vi "ecg_ncs_v8_67.vi"() -> ()   [LabVIEW 2016]
uses:
  <instrlib>/niUSRP/niUSRP Timestamp.ctl
  C:/Program Files/National Instruments/LabVIEW 2016/examples/Instrument IO/Serial/support/Serial - Settings.ctl
  State.ctl
  <vilib>/Instr/_visa.llb/VISA Configure Serial Port (Instr).vi
  <instrlib>/niUSRP/niUSRP Fetch Rx Data (2D CDB).vi
  <instrlib>/niUSRP/niUSRP Write Tx Data (2D CDB).vi
panel:
  out "size(s) 3":i32
  out "AmpNcsDSLast":dbl[](array[numeric])
  in  "Low-Pass Freq":dbl=200.0 format="%#_13g"
  in  "Wait  ECG":i32=1
  in  "max queue size":i32=-1
  in  "Wait NCS":i32=-1
  out "ECG time":u32
  out "NCS time":u32
  in  "File Name 3":string="Test2"
  out "size(s) 4":i32
  in  "maxWrite 2":i32=2000
  out "AmpNcs":dbl[](array[numeric])
  out "PhNcs":dbl[](array[numeric])
  in  "Sampling Rate":i32=500
  out "AmpNcsDS":dbl[](array[numeric])
  out "PhNcsDS":dbl[](array[numeric])
  in  "Tab Control 3":enum32{"ECG Sample", "ECG"}(tab)
  out "?":i32(graph)
  out "?":i16(graph)
  in  "maxWrite":i32=2000
  out "size(s) 2":i32
  out "sizeNcsDS":i32
  in  "File Name":string="freq2G_1"
  in  "Path":path=path "D:/Research/SummerFall17Spring18/CnC/NCS/EcgNcsCorrelation/CodeAndData/Data/Mar03"
  out "#Loop = #Packets Received":i32
  out "ECGsample":i16
  out "error IO 2":errorcluster={"status"=FALSE, "code"=-1074118647, "source"=""}
  in  "Serial Settings":T1={"baud rate"=57600, "data bits"=8, "parity"=enum."None", "stop bits"=10, "flow control"=0} {"flow control" items=["None"=0, "XON/XOFF"=1, "RTS/CTS"=2, "DTR/DSR"=4]; "stop bits" items=["1.0"=10, "1.5"=15, "2.0"=20]; "data bits" min=5 max=8 step=1; "baud rate" items=["75"=75, "110"=110, "134"=134, "150"=150, "300"=300, "600"=600, "1200"=1200, "1800"=1800, "2400"=2400, "4800"=4800, "7200"=7200, "9600"=9600, "14400"=14400, "19200"=19200, "28800"=28800, "38400"=38400, "56000"=56000, "57600"=57600, "115200"=115200, "128000"=128000, "230400"=230400]}
  in  "VISA resource name":refnum<visa-resource-name>="bmd101"
  in  "byte count":u32=1
  out "Coerced Rx IQ Rate":dbl
  out "Gain":dbl=-15.0
  out "Bandwidth":dbl=56000000.0
  out "Coerced Carrier Frequency":dbl=2000000000.0 format="%#.17g"
  out "Coerced Tx IQ rate":dbl=1000000.0
  out "error IO":errorcluster={"status"=FALSE, "code"=-1074118647, "source"=""}
  in  "Rx Number of Samples":i32=10000
  in  "Tab Control 2":enum32{"NI-294x/295x", "NI-2900/2901"}(tab)=enum."NI-2900/2901"
  in  "Rx carrier frequency [Hz]":dbl=2000000000.0 format="%#_6p"
  in  "Tx carrier frequency [Hz]":dbl=1000000000.0 format="%#_6p"
  in  "Start Trigger Time":T2={"whole seconds"=1, "fractional seconds"=0.0}
  in  "Tab Control":T3(tab)
  out "?":dbl[](graph)
  out "NCS Amp Chart":dbl[](graph)=[0.011967714738528729, 0.012021355192189592, 0.012015275039596582, 0.011969166030167903, 0.011958890166168242, 0.012007893820858737, 0.012022893722444085, 0.011978222225113794, 0.011969989939463181, 0.012003099640895068]
  out "NCS Phase Chart":dbl[](graph)=[0.011967714738528729, 0.012021355192189592, 0.012015275039596582, 0.011969166030167903, 0.011958890166168242, 0.012007893820858737, 0.012022893722444085, 0.011978222225113794, 0.011969989939463181, 0.012003099640895068]
  out "Tx Waveform Graph":waveform(dbl)[](graph)
  in  "Stop":bool
  in  "Tone Amplitude":dbl=0.707 step=0.05 format="%#.6g"
  in  "Tone  Frequency":dbl=5000.0 format="%#_6p"
  in  "Tx Waveform Size":dbl=2000.0
  in  "Device Name":refnum<k15>="MyB210"
  in  "Tx Gain":dbl=28.0 format="%#_6f"
  in  "Tx IQ Rate":dbl=1000000.0 format="%#_6p"
  in  "Rx Gain":dbl=32.0 format="%#_6f"
  in  "Rx IQ Rate":dbl=1000000.0 format="%#_6p"
  # "Rx Settings"
  # "Tx Settings"
  # "Note that on the NI-2900 and NI-2901, both Rx channels share an LO and both Tx channels share an LO. However, on the NI-294x/295x devices, Rx and Tx of channel 0 share an LO and Rx and Tx of channel 1 share an LO."
  # "Rx: Number of samples should be 1e6/512 in one loop."
  # "This Tx graph should always have end and start tied up since this is being sent in a loop continuously. Otherwise phase jumps will be noticed."
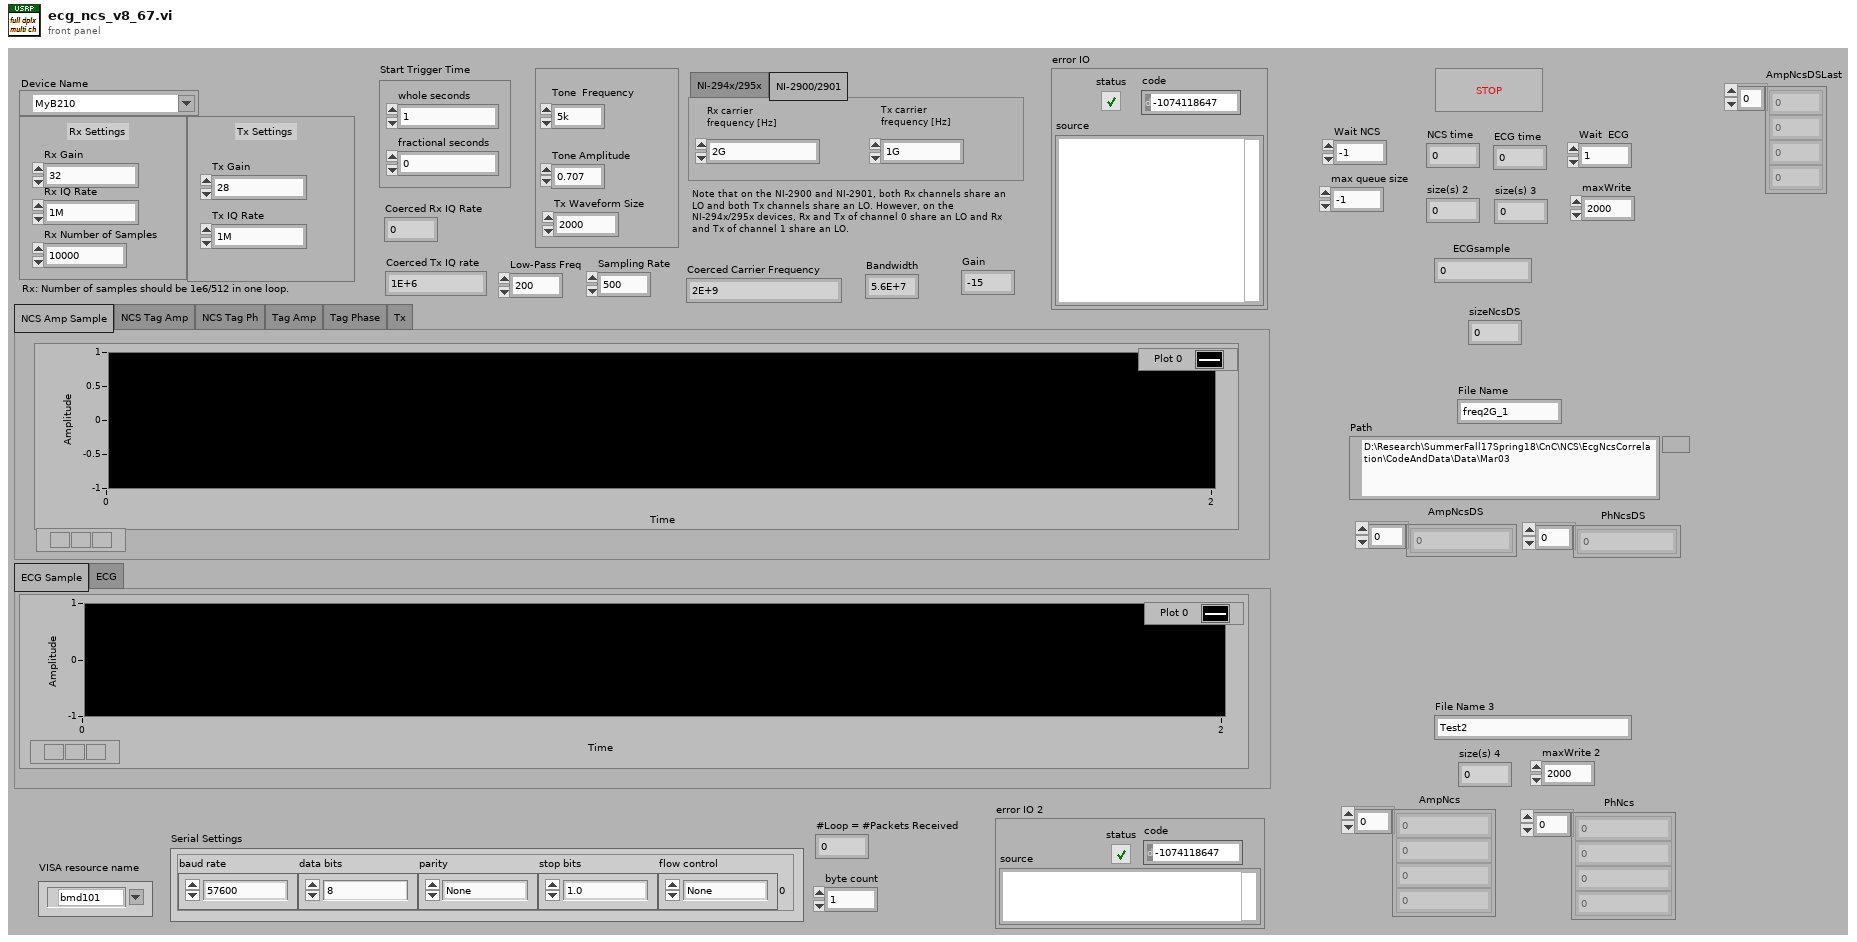
[diagram p1: front panel]
types:
  T1 = typedef "Serial - Settings.ctl" = cluster{"baud rate":u32, "data bits":u16, "parity":enum16{"None", "Odd", "Even", "Mark", "Space"}, "stop bits":u16, "flow control":u16}
  T2 = typedef "niUSRP Timestamp.ctl" = cluster{"whole seconds":u64, "fractional seconds":dbl}
  T3 = enum32{"NCS Amp Sample", "NCS Tag Amp", "NCS Tag Ph", "Tag Amp", "Tag Phase", "Tx"}
  T4 = typedef "State.ctl" = enum16{"Initialize", "get byte", "check", "packet received", "packet approved"}
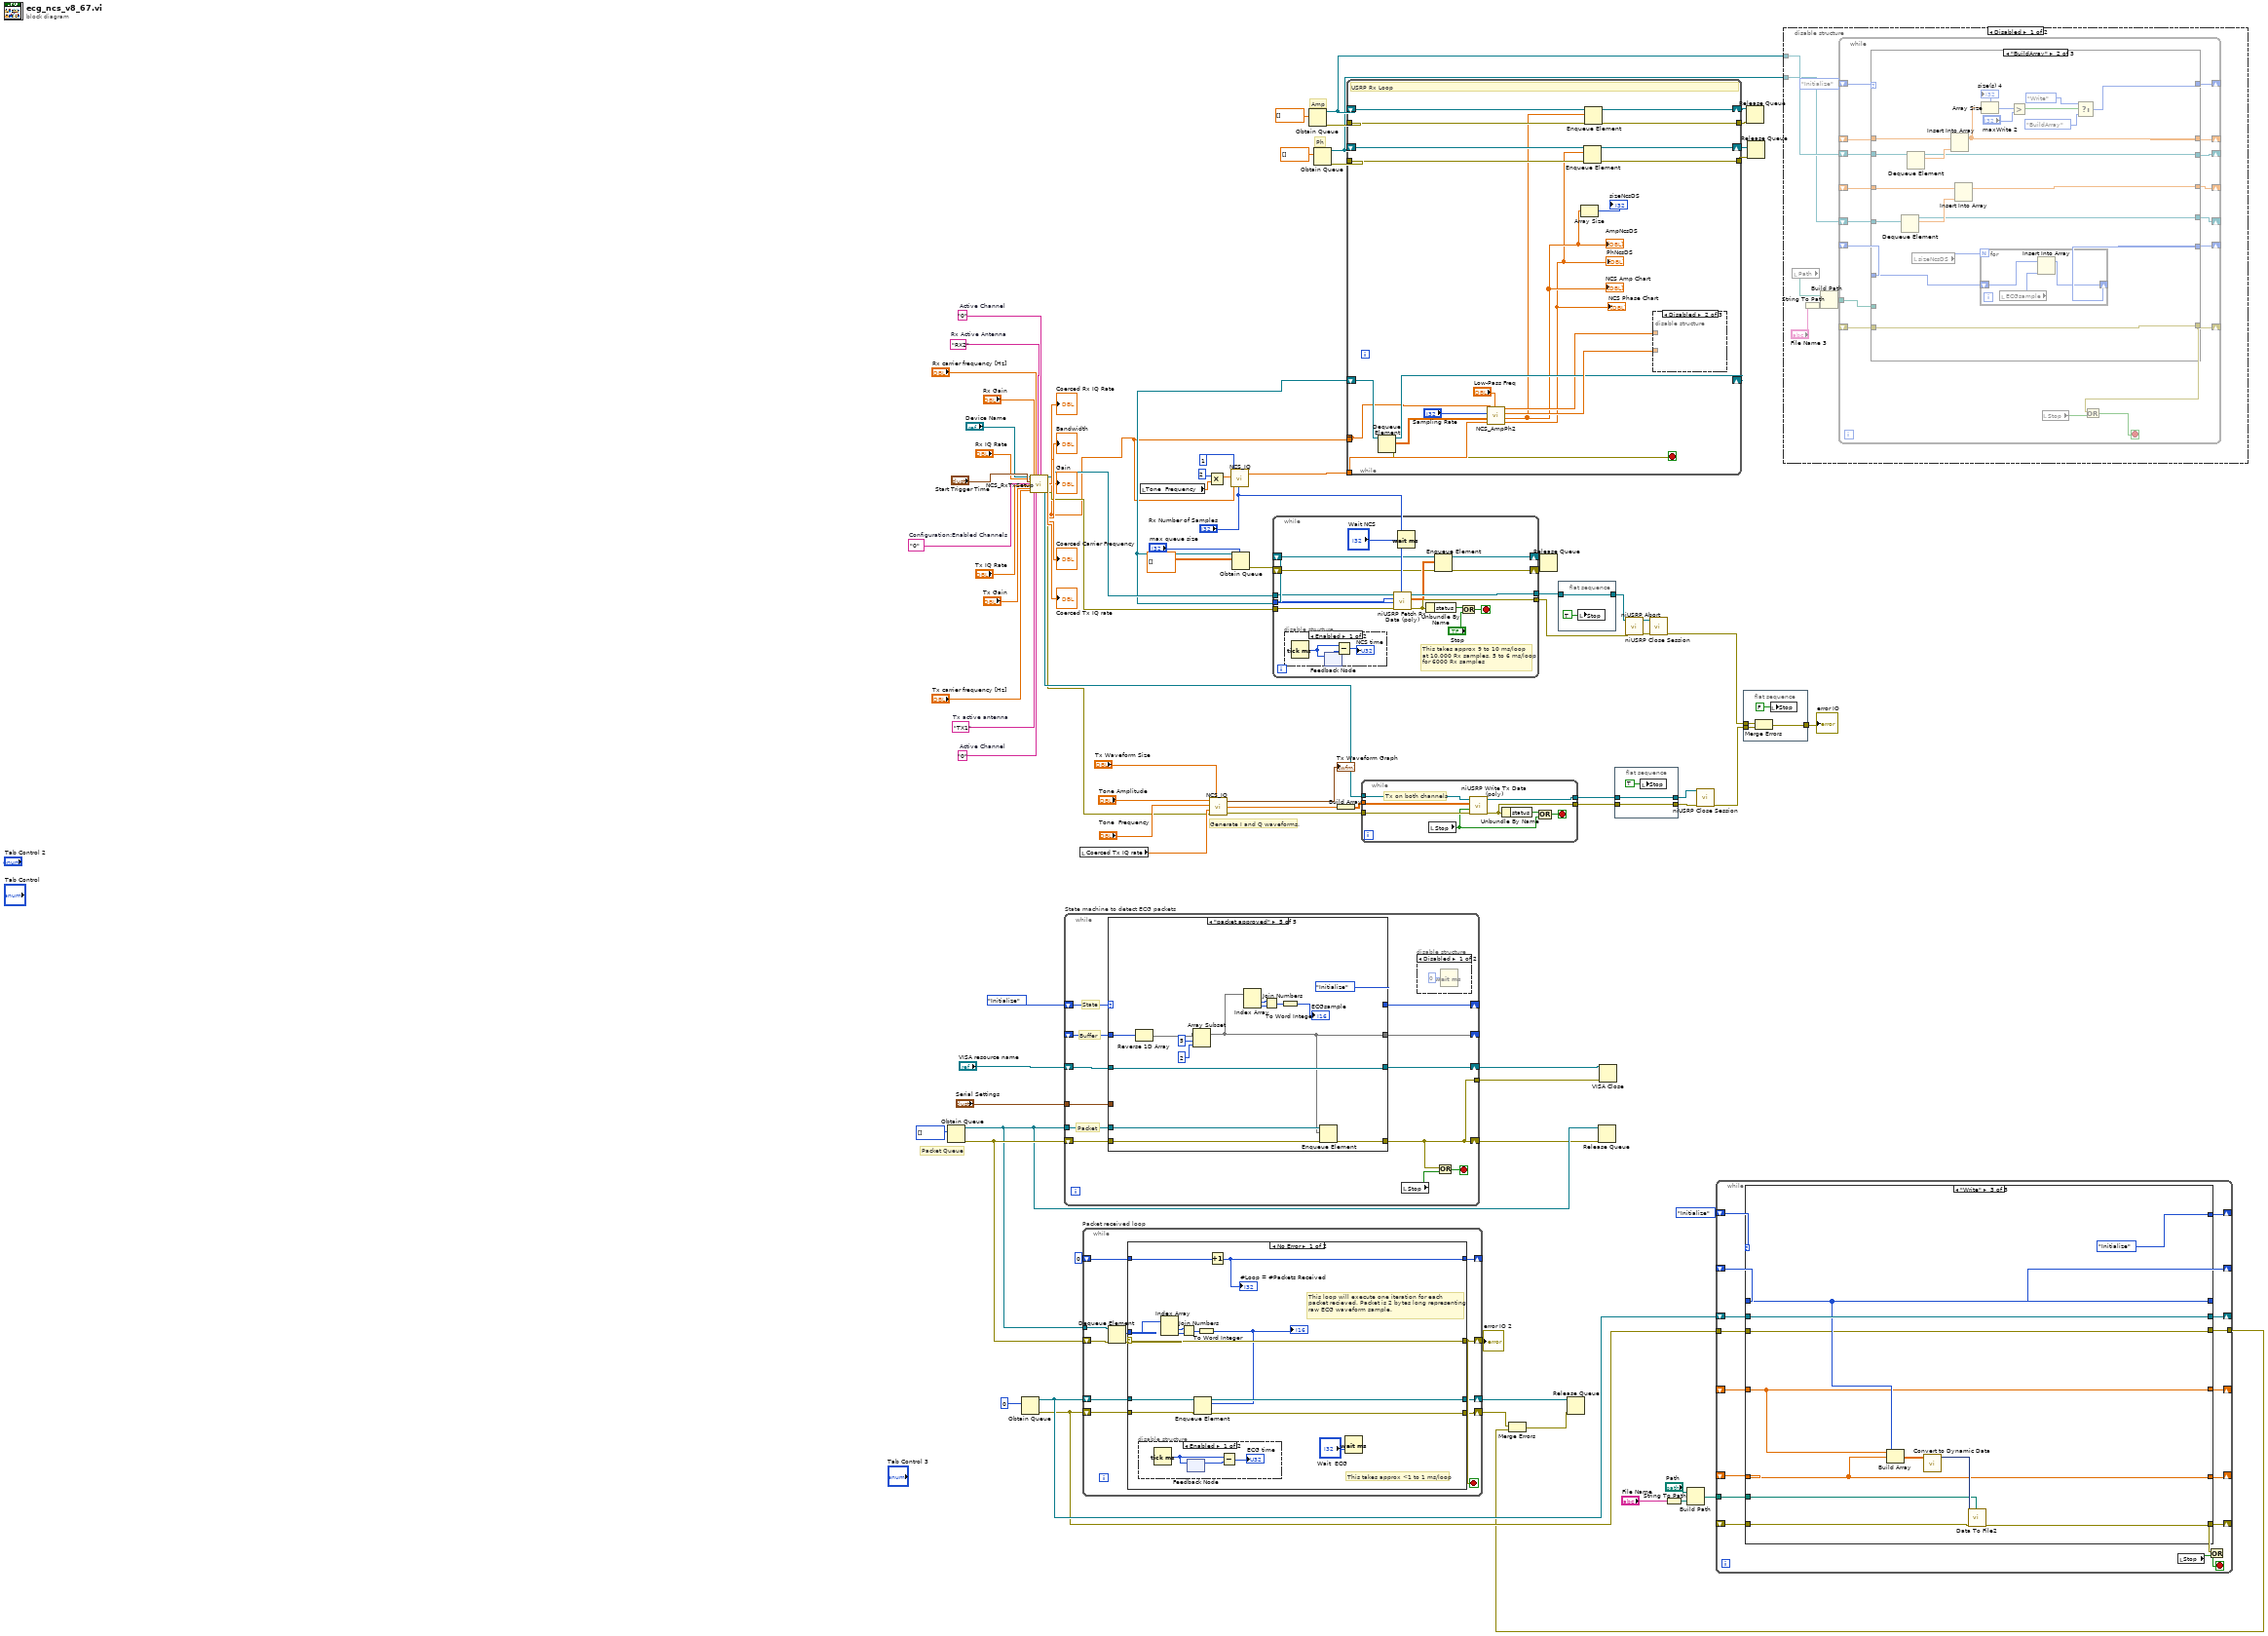
[diagram p0: block diagram]
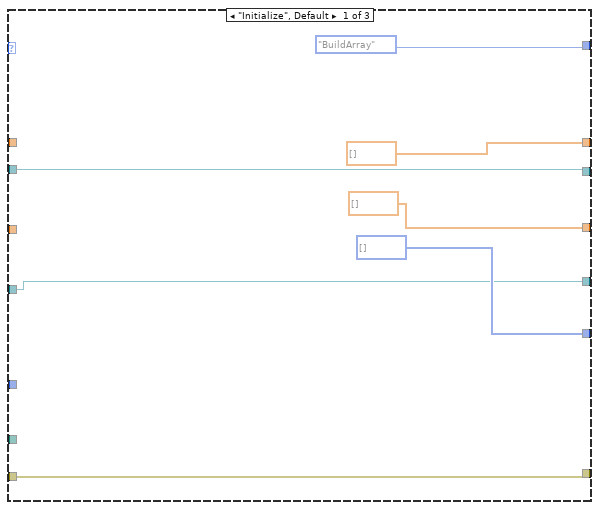
[diagram p2: hidden frame]
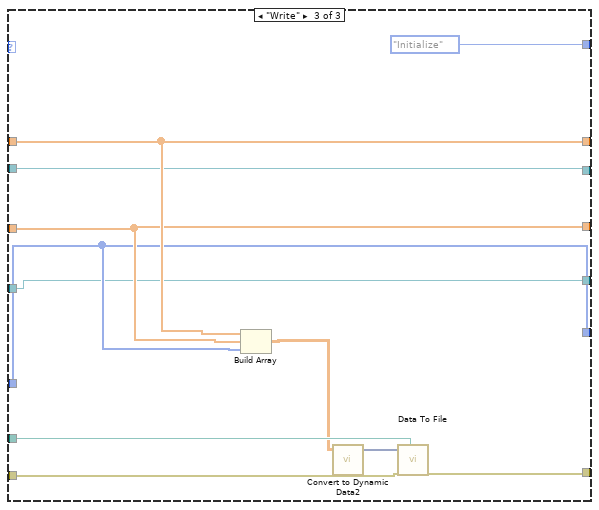
[diagram p3: hidden frame]
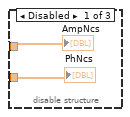
[diagram p5: hidden frame]
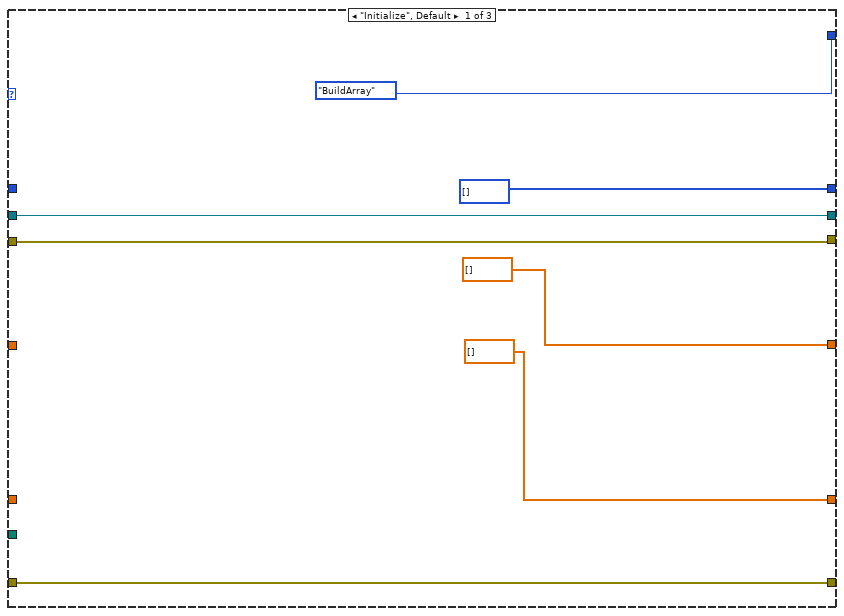
[diagram p7: hidden frame]
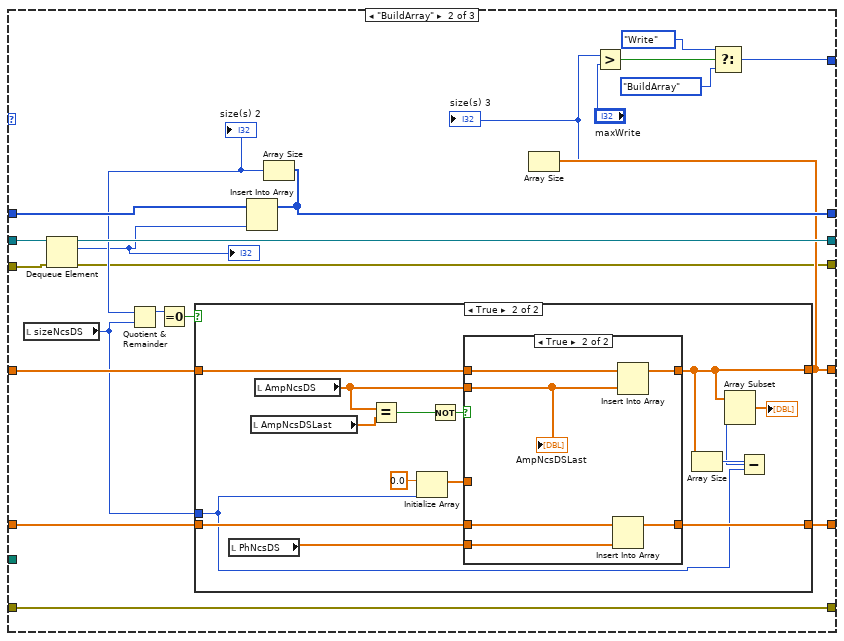
[diagram p8: hidden frame]
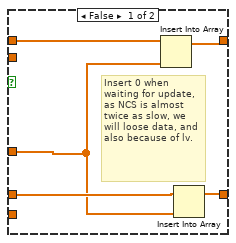
[diagram p10: hidden frame]
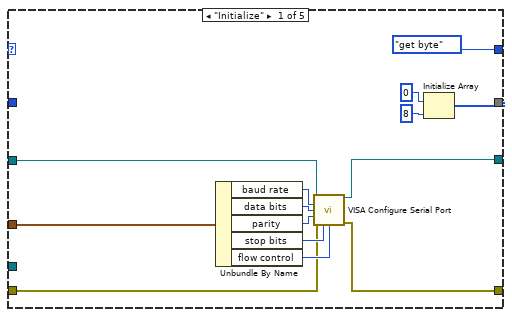
[diagram p15: hidden frame]
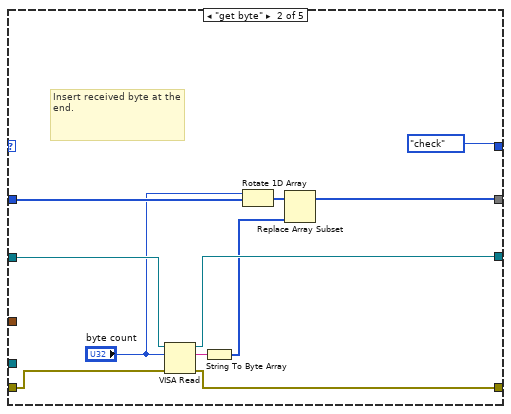
[diagram p16: hidden frame]
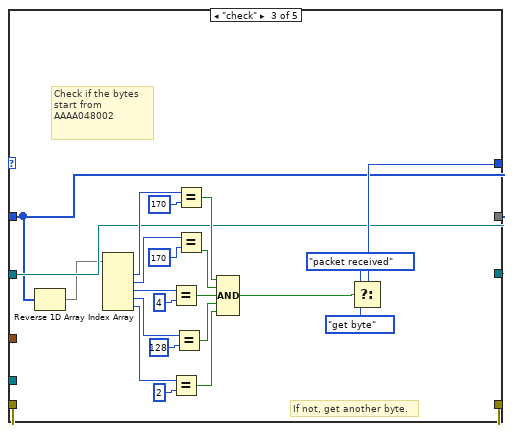
[diagram p17: hidden frame]
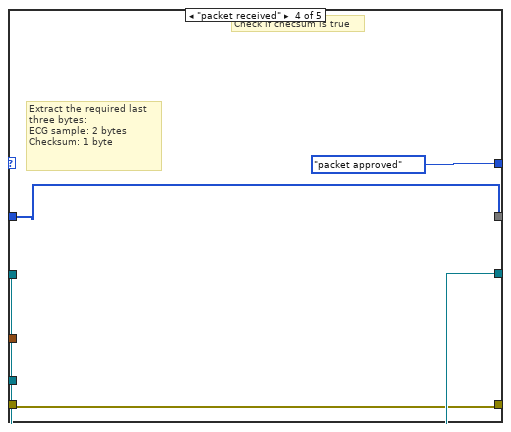
[diagram p18: hidden frame]
diagram:
  w49 = "0"  # Active Channel
  w50 = "0"  # Active Channel
  w79 = "RX2"  # Rx Active Antenna
  w75 = "TX1"  # Tx active antenna
  w64 = "0"  # Configuration:Enabled Channels
  # "Ph"
  # "Amp"
  # "Packet Queue"
  # "Generate I and Q waveforms."
  n1 = Obtain Queue(element data type=u8[] []) -> (queue out=w45:refnum<queue>, error out=w46:errorcluster)  [unwired: 4 in, 1 out]
  n2 = Obtain Queue(element data type=0) -> (queue out=w19:refnum<queue>, error out=w5:errorcluster)  [unwired: 4 in, 1 out]
  n3 = call "NCS_RxTxSetup.vi"("IVI Refnum in"="Device Name", "Rx IQ Rate"="Rx IQ Rate", "Start Trigger Time"="Start Trigger Time", "Configuration:Enabled Channels"=w64, "Tx IQ Rate"="Tx IQ Rate", "Tx Gain"="Tx Gain", "Tx carrier frequency [Hz]"="Tx carrier frequency [Hz]", "Rx Gain"="Rx Gain", "Tx active antenna"=w75, "Rx carrier frequency [Hz]"="Rx carrier frequency [Hz]", "Active Channel"=w49, "Rx Active Antenna"=w79, "Active Channel 2"=w50) -> ("session handle out"=w86:refnum<k15>, "IVI Refnum out"=w35:refnum<k15>, "Coerced Rx IQ Rate"=w7:dbl, "Bandwidth"=→"Bandwidth":dbl, "Gain"=→"Gain":dbl, "Carrier Frequency"=→"Coerced Carrier Frequency":dbl, "IQ Rate 2"=→"Coerced Tx IQ rate":dbl, "error out"=w36:errorcluster)  [unwired: 7 in]
  "Coerced Rx IQ Rate" <- w7
  n4 = while "State machine to detect ECG packets" {
    shift-right: [w89] -> w40
    shift-left: w46 -> [w95]
    shift-right: [w98] -> _
    shift-left: State."Initialize" ("State") -> [w97]
    shift-right: [w94] -> _
    shift-left: _ -> [w96]
    tunnel: w45 -> [w93]
    shift-right: [w92] -> w41
    shift-left: "VISA resource name" -> [w91]
    tunnel: "Serial Settings" -> [w90]
    tunnel: [w89] -> w39
    stop <- w88 stop-if-true
    # "State"
    # "Buffer"
    # "Packet"
    n5 = case shown="\"packet approved\"" w97 {
      tunnel: [w110 w122 w126 w149 w153] -> w94
      tunnel: [State."get byte" ("State") State."check" ("f") w146 State."packet approved" ("State") State."Initialize" ("State")] -> w98
      tunnel: w96 -> [_ w115 w126 w149 w158]
      tunnel: w95 -> [w104 w119 w147 w150 w161]
      tunnel: [w103 w118 w147 w150 w160] -> w89
      tunnel: w93 -> [_ _ _ _ w162]
      tunnel: [w102 w120 w127 w151 w159] -> w92
      tunnel: w91 -> [w101 w121 w127 w151 w159]
      tunnel: w90 -> [w100 _ _ _ _]
      frame "Initialize" {
        n6 = Unbundle By Name(w100) -> ("baud rate"=w109:u32, "data bits"=w108:u16, "parity"=w107:enum16{"None", "Odd", "Even", "Mark", "Space"}, "stop bits"=w106:u16, "flow control"=w105:u16)
        n7 = call-poly "VISA Configure Serial Port"("VISA resource name"=w101, "baud rate (9600)"=w109, "data bits (8)"=w108, "parity (0:none)"=w107, "error in (no error)"=w104, "stop bits (10: 1 bit)"=w106, "flow control (0:none)"=w105) -> ("VISA resource name out"=w102:refnum<visa-resource-name>, "error out"=w103:errorcluster)  [unwired: 3 in, 4 out]
        n8 = Initialize Array(u8 0, 8 ("dimension size")) -> (w110:u8[])
      }
      frame "get byte" {
        # "Insert received byte at the end."
        n9 = VISA Read(VISA resource name=w121, byte count="byte count", error in (no error)=w119) -> (VISA resource name out=w120:refnum<visa-resource-name>, read buffer=w117:string, error out=w118:errorcluster)  [unwired: 1 out]
        n10 = String To Byte Array(string=w117) -> (unsigned byte array=w116:u8[])
        n11 = Rotate 1D Array(1:w115, 2:"byte count") -> (0:w123:u8[])
        n12 = Replace Array Subset(array=w123, new element=w116) -> (w122:u8[])  [unwired: 1 in]
      }
      frame "check" {
        # "If not, get another byte."
        # "Check if the bytes start from AAAA048002"
        n13 = Reverse 1D Array(array=w126) -> (reversed array=w125:u8[])
        n14 = Index Array(array=w125) -> (element #1=w133:u8, element #2=w132:u8, element #3=w131:u8, element #4=w130:u8, element #5=w129:u8)  [unwired: 5 in]
        n15 = Equal?(x=w131, y=u8 4 ("element")) -> (x = y?=w136:bool)
        n16 = Equal?(x=w129, y=u8 2 ("element")) -> (x = y?=w134:bool)
        n17 = Equal?(x=w130, y=u8 128 ("element")) -> (x = y?=w135:bool)
        n18 = Equal?(x=w133, y=u8 170 ("element")) -> (x = y?=w138:bool)
        n19 = Equal?(x=w132, y=u8 170 ("element")) -> (x = y?=w137:bool)
        n20 = Compound Arithmetic op=AND(w138, w137, w136, w135, w134) -> (w128:bool)
        n21 = Select(t=State."packet received" ("f"), s=w128, f=State."get byte") -> (s? t:f=w146:T4)
      }
      frame "packet received" {
        # "Check if checsum is true"
        # "Extract the required last three bytes: \nECG sample: 2 bytes\nChecksum: 1 byte"
      }
      frame "packet approved" {
        n22 = Reverse 1D Array(array=w158) -> (reversed array=w157:u8[])
        n23 = Array Subset(array=w157, index=5, length=2 ("index")) -> (w153:u8[])
        n24 = Index Array(array=w153) -> (element #1=w156:u8, element #2=w155:u8)  [unwired: 2 in]
        n25 = Join Numbers(hi=w156, lo=w155) -> ((hi.lo)=w154:u16)
        n26 = To Word Integer(number=w154) -> (16bit integer=→"ECGsample":i16)
        n27 = Enqueue Element(queue=w162, element=w153, error in (no error)=w161) -> (error out=w160:errorcluster)  [unwired: 1 in, 2 out]
      }
    }
    n28 = local read "Stop"() -> (w87:bool)
    n29 = disable-structure shown="Disabled" {
      frame Disabled {
        n30 = Wait (ms)(milliseconds to wait=u32 0) -> ()  [unwired: 1 out]
      }
      frame Enabled {
      }
    }
    n31 = Or(x=w89, y=w87) -> (x .or. y?=w88:bool)
  }
  n32 = local read "Coerced Tx IQ rate"() -> (w59:dbl)
  n33 = while "Packet received loop" {
    shift-right: [w172] -> w42
    shift-left: w46 -> [w176]
    tunnel: w45 -> [w175]
    shift-right: [w170] -> _
    shift-left: 0 -> [w171]
    shift-right: [w167] -> w20
    shift-left: w19 -> [w169]
    shift-right: [w166] -> w4
    shift-left: w5 -> [w168]
    stop <- w172 stop-if-true
    n34 = Dequeue Element(queue=w175, error in (no error)=w176) -> (element=w174:u8[], error out=w173:errorcluster)  [unwired: 1 in, 2 out]
    n35 = case shown="No Error" w173 {
      selector: w173 -> [w183 w196]
      tunnel: w174 -> [w189 _]
      tunnel: [w183 w196] -> w172
      tunnel: w171 -> [w185 w195]
      tunnel: [w184 w195] -> w170
      tunnel: w169 -> [w182 w194]
      tunnel: w168 -> [w181 w193]
      tunnel: [w180 w194] -> w167
      tunnel: [w179 w193] -> w166
      frame No Error {
        # "This takes approx <1 to 1 ms/loop"
        # "This loop will execute one iteration for each\npacket recieved. Packet is 2 bytes long representing \nraw ECG waveform sample."
        n36 = disable-structure shown="Enabled" {
          frame Enabled {
            n37 = Tick Count (ms)() -> (millisecond timer value=w192:u32)
            n38 = feedback #1() -> (w191:u32)  [unwired: 1 in]
            n39 = feedback-in #1(w192) -> ()
            n40 = Subtract(x=w192, y=w191) -> (x-y=→"ECG time":u32)
          }
          frame Disabled {
          }
        }
        n41 = Index Array(array=w189) -> (element #1=w188:u8, element #2=w187:u8)  [unwired: 2 in]
        n42 = Join Numbers(hi=w188, lo=w187) -> ((hi.lo)=w186:u16)
        n43 = To Word Integer(number=w186) -> (16bit integer=w178:i16)
        "?" <- w178
        n44 = Enqueue Element(queue=w182, element=w178, error in (no error)=w181) -> (queue out=w180:refnum<queue>, error out=w179:errorcluster)  [unwired: 1 in, 1 out]
        n45 = Increment(x=w185) -> (x+1=w184:i32)
        "#Loop = #Packets Received" <- w184
        n46 = Wait (ms)(milliseconds to wait="Wait  ECG") -> ()  [unwired: 1 out]
      }
      frame Error {
      }
    }
  }
  "error IO 2" <- w42
  n47 = local read "Tone  Frequency"() -> (w63:dbl)
  n48 = Multiply(x=2, y=w63) -> (x*y=w28:dbl)
  n49 = call "NCS_IQ.vi"("Tone Amplitude"="Tone Amplitude", "Waveform Size"="Tx Waveform Size", "Tone Frequency"="Tone  Frequency", "Coerced IQ rate"=w59, "error in (no error)"=w36) -> ("IQ waveform"=→"Tx Waveform Graph":waveform(dbl)[], "IQ waveform array"=w57:cdb[], "error out"=w58:errorcluster)  [unwired: 1 in]
  n50 = call "NCS_IQ.vi"("Tone Amplitude"=1, "Waveform Size"="Rx Number of Samples", "Tone Frequency"=w28, "Coerced IQ rate"=w7) -> ("IQ waveform array"=w6:cdb[])  [unwired: 2 in, 2 out]
  n51 = Obtain Queue(max queue size (-1, unlimited)="max queue size", element data type=dbl[][] []) -> (queue out=w8:refnum<queue>, error out=w32:errorcluster)  [unwired: 3 in, 1 out]
  n52 = while {
    tunnel: w36 -> [w210]
    tunnel: w35 -> [w209]
    tunnel: [w208] -> w34
    tunnel: [w200] -> w33
    shift-right: [w204] -> w31
    shift-left: w32 -> [w205]
    shift-right: [w203] -> w30
    shift-left: w8 -> [w207]
    tunnel: "Rx Number of Samples" -> [w202]
    stop <- w199 stop-if-true
    # "This takes approx 9 to 10 ms/loop\nat 10,000 Rx samples, 5 to 6 ms/loop \nfor 6000 Rx samples"
    n53 = disable-structure shown="Enabled" {
      frame Enabled {
        n54 = Tick Count (ms)() -> (millisecond timer value=w213:u32)
        n55 = feedback #2() -> (w212:u32)  [unwired: 1 in]
        n56 = feedback-in #2(w213) -> ()
        n57 = Subtract(x=w213, y=w212) -> (x-y=→"NCS time":u32)
      }
      frame Disabled {
      }
    }
    n58 = call-poly <instrlib>:"niUSRP Fetch Rx Data (poly).vi"("session handle"=w209, "number of samples"=w202, "error in (no error)"=w210) -> ("session handle out"=w208:refnum<k15>, "data"=w206:cdb[][], "error out"=w200:errorcluster)  [unwired: 9 in, 1 out]
    n59 = Wait (ms)(milliseconds to wait="Wait NCS") -> ()  [unwired: 1 out]
    n60 = Unbundle By Name(w200) -> ("status"=w201:bool)
    n61 = Enqueue Element(queue=w207, element=w206, error in (no error)=w205) -> (queue out=w203:refnum<queue>, error out=w204:errorcluster)  [unwired: 1 in, 1 out]
    n62 = Or(x=w201, y="Stop") -> (x .or. y?=w199:bool)
  }
  n63 = Obtain Queue(element data type=dbl[] []) -> (queue out=w10:refnum<queue>, error out=w17:errorcluster)  [unwired: 4 in, 1 out]
  n64 = Obtain Queue(element data type=dbl[] []) -> (queue out=w9:refnum<queue>, error out=w11:errorcluster)  [unwired: 4 in, 1 out]
  n65 = Build Array(w57) -> (w83:cdb[][])
  n66 = while {
    tunnel: [w218] -> _
    shift-right: [w231] -> _
    shift-left: w8 -> [w232]
    tunnel: w6 -> [w229]
    shift-right: [w223] -> w16
    shift-left: w10 -> [w224]
    tunnel: w17 -> [w227]
    tunnel: [w226] -> w15
    shift-right: [w221] -> w13
    shift-left: w9 -> [w222]
    tunnel: [w220] -> w12
    tunnel: w11 -> [w219]
    tunnel: w7 -> [w218]
    stop <- w228 stop-if-true
    # "USRP Rx Loop"
    n67 = Dequeue Element(queue=w232) -> (queue out=w231:refnum<queue>, element=w230:dbl[][], error out=w228:errorcluster)  [unwired: 2 in, 1 out]
    n68 = call "NCS_AmpPh2.vi"("Low-Pass Freq"="Low-Pass Freq", "IQ"=w229, "data"=w230, "Sampling Rate"="Sampling Rate", "Coerced Rx IQ Rate"=w218) -> ("Phase DownSampled"=w215:dbl[], "Amp DownSampled"=w216:dbl[], "Phase"=w233:dbl[], "Amplitude"=w225:dbl[])  [unwired: 2 in, 1 out]
    "AmpNcsDS" <- w216
    "PhNcsDS" <- w215
    "NCS Amp Chart" <- w216
    "NCS Phase Chart" <- w215
    n69 = Array Size(array=w216) -> (size(s)=→"sizeNcsDS":i32)
    n70 = Enqueue Element(queue=w222, element=w215, error in (no error)=w219) -> (queue out=w221:refnum<queue>, error out=w220:errorcluster)  [unwired: 1 in, 1 out]
    n71 = Enqueue Element(queue=w224, element=w216, error in (no error)=w227) -> (queue out=w223:refnum<queue>, error out=w226:errorcluster)  [unwired: 1 in, 1 out]
    n72 = disable-structure shown="Disabled" {
      disable-tunnel: w225 -> [w235 _ _]
      disable-tunnel: w233 -> [w236 _ _]
      frame Disabled {
        "AmpNcs" <- w235
        "PhNcs" <- w236
      }
      frame Disabled {
      }
      frame Enabled {
      }
    }
  }
  n73 = while {
    tunnel: w86 -> [w244]
    tunnel: w58 -> [w243]
    tunnel: [w241] -> w74
    tunnel: [w239] -> w70
    tunnel: w83 -> [w237]
    stop <- w240 stop-if-true
    # "Tx on both channels"
    n74 = local read "Stop"() -> (w238:bool)
    n75 = call-poly <instrlib>:"niUSRP Write Tx Data (poly).vi"("session handle"=w244, "data"=w237, "end of data?"=w238, "error in (no error)"=w243) -> ("session handle out"=w239:refnum<k15>, "error out"=w241:errorcluster)  [unwired: 10 in]
    n76 = Unbundle By Name(w241) -> ("status"=w242:bool)
    n77 = Compound Arithmetic op=OR(w242, w238) -> (w240:bool)
  }
  n78 = Release Queue(queue=w30, error in (no error)=w31) -> ()  [unwired: 1 in, 3 out]
  n79 = flat-sequence {
    tunnel: [w245] -> w72
    tunnel: w34 -> [w245]
    frame #0 {
      n80 = local write "Stop"(TRUE ("STOP")) -> ()
    }
  }
  n81 = Release Queue(queue=w45, error in (no error)=w40) -> ()  [unwired: 1 in, 3 out]
  n82 = VISA Close(VISA resource name=w41, error in (no error)=w39) -> ()  [unwired: 1 out]
  n83 = flat-sequence {
    tunnel: [w248] -> w73
    tunnel: w74 -> [w248]
    tunnel: [w247] -> w71
    tunnel: w70 -> [w247]
    frame #0 {
      n84 = local write "Stop"(TRUE ("STOP")) -> ()
    }
  }
  n85 = call <instrlib>:"niUSRP Abort.vi"("session handle"=w72, "error in (no error)"=w33) -> ("session handle out"=w85:refnum<k15>, "error out"=w84:errorcluster)  [unwired: 12 in]
  n86 = call <instrlib>:"niUSRP Close Session.vi"("session handle"=w85, "error in (no error)"=w84) -> ("error out"=w67:errorcluster)  [unwired: 13 in]
  n87 = String To Path(string="File Name") -> (path=w26:path)
  n88 = Build Path(base path="Path", name or relative path=w26) -> (appended path=w22:path)
  n89 = call <instrlib>:"niUSRP Close Session.vi"("session handle"=w71, "error in (no error)"=w73) -> ("error out"=w69:errorcluster)  [unwired: 13 in]
  n90 = while {
    shift-right: [w265] -> _
    shift-left: _ -> [w266]
    shift-right: [w263] -> _
    shift-left: _ -> [w264]
    shift-right: [w261] -> _
    shift-left: enum16{"Initialize", "BuildArray", "Write"}."Initialize" -> [w262]
    tunnel: w22 -> [w260]
    shift-right: [w257] -> _
    shift-left: _ -> [w256]
    shift-right: [w254] -> _
    shift-left: w19 -> [w255]
    shift-right: [w253] -> _
    shift-left: _ -> [w252]
    tunnel: w5 -> [w251]
    tunnel: [w250] -> w3
    stop <- w258 stop-if-true
    n91 = case shown="\"Write\"" w262 {
      tunnel: w266 -> [_ w295 w327]
      tunnel: [i32[] [] w293 w327] -> w265
      tunnel: w264 -> [_ w294 w325]
      tunnel: [dbl[] [] w283 w325] -> w263
      tunnel: [enum16{"Initialize", "BuildArray", "Write"}."BuildArray" w288 enum16{"Initialize", "BuildArray", "Write"}."Initialize"] -> w261
      tunnel: w260 -> [_ _ w332]
      tunnel: [w272 w287 w330] -> w257
      tunnel: w256 -> [w272 w287 w329]
      tunnel: w255 -> [w271 w286 w328]
      tunnel: [w271 w285 w328] -> w254
      tunnel: [dbl[] [] w279 w326] -> w253
      tunnel: w252 -> [_ w284 w326]
      tunnel: w251 -> [w267 w276 w324]
      tunnel: [w267 w275 w324] -> w250
      frame "Initialize", Default {
      }
      frame "BuildArray" {
        n92 = local read "sizeNcsDS"() -> (w274:i32)
        n93 = Dequeue Element(queue=w286, error in (no error)=w276) -> (queue out=w285:refnum<queue>, element=w277:i32, error out=w275:errorcluster)  [unwired: 1 in, 1 out]
        "?" <- w277
        n94 = Insert Into Array(array=w295, new element=w277) -> (w293:i32[])  [unwired: 1 in]
        n95 = Array Size(array=w293) -> (size(s)=w282:i32)
        "size(s) 2" <- w282
        n96 = Quotient & Remainder(x=w282, y=w274) -> (x-y*floor(x/y)=w281:i32)  [unwired: 1 out]
        n97 = Equal To 0?(x=w281) -> (x = 0?=w280:bool)
        n98 = case shown="True" w280 {
          tunnel: w294 -> [w296 w312]
          tunnel: [w296 w311] -> w283
          tunnel: w284 -> [w297 w309]
          tunnel: [w297 w303] -> w279
          tunnel: w274 -> [_ w299]
          frame False {
          }
          frame True {
            n99 = local read "PhNcsDS"() -> (w310:dbl[])
            n100 = local read "AmpNcsDSLast"() -> (w298:dbl[])
            n101 = local read "AmpNcsDS"() -> (w308:dbl[])
            n102 = Equal?(x=w308, y=w298) -> (x = y?=w307:bool)
            n103 = Initialize Array(0.0 ("element"), w299) -> (w304:dbl[])
            n104 = Not(x=w307) -> (.not. x?=w306:bool)
            n105 = case shown="True" w306 {
              tunnel: w309 -> [w317 w323]
              tunnel: w312 -> [w315 w322]
              tunnel: [w314 w321] -> w311
              tunnel: w310 -> [_ w320]
              tunnel: w308 -> [_ w319]
              tunnel: [w316 w318] -> w303
              tunnel: w304 -> [w313 _]
              frame False {
                # "Insert 0 when \nwaiting for update,\nas NCS is almost \ntwice as slow, we \nwill loose data, and also because of lv."
                n106 = Insert Into Array(array=w317, new element=w313) -> (w316:dbl[])  [unwired: 1 in]
                n107 = Insert Into Array(array=w315, new element=w313) -> (w314:dbl[])  [unwired: 1 in]
              }
              frame True {
                n108 = Insert Into Array(array=w322, new element=w320) -> (w321:dbl[])  [unwired: 1 in]
                n109 = Insert Into Array(array=w323, new element=w319) -> (w318:dbl[])  [unwired: 1 in]
                "AmpNcsDSLast" <- w319
              }
            }
            n110 = Array Size(array=w303) -> (size(s)=w302:i32)
            n111 = Subtract(x=w302, y=w299) -> (x-y=w300:i32)
            n112 = Array Subset(array=w303, index=w300) -> (→"?":dbl[])  [unwired: 1 in]
          }
        }
        n113 = Array Size(array=w279) -> (size(s)=w278:i32)
        "size(s) 3" <- w278
        n114 = Greater?(x=w278, y="maxWrite") -> (0:w291:bool)
        n115 = Select(t=enum16{"Initialize", "BuildArray", "Write"}."Write", s=w291, f=enum16{"Initialize", "BuildArray", "Write"}."BuildArray") -> (s? t:f=w288:enum16{"Initialize", "BuildArray", "Write"})
      }
      frame "Write" {
        n116 = Build Array(w326, w325, w327) -> (w331:dbl[][])
        n117 = call "Convert to Dynamic Data"("2D Array"=w331) -> ("Dynamic Data Type"=w333:dynamicdata)  [unwired: 3 in]
        n118 = call "Data To File2"("Signals"=w333, "error in (no error)"=w329, "Filename"=w332) -> ("error out"=w330:errorcluster)  [unwired: 14 in, 2 out]
      }
    }
    n119 = local read "Stop"() -> (w259:bool)
    n120 = Or(x=w257, y=w259) -> (x .or. y?=w258:bool)
  }
  n121 = Merge Errors(w4, w3) -> (w2:errorcluster)
  n122 = Release Queue(queue=w20, error in (no error)=w2) -> ()  [unwired: 1 in, 3 out]
  n123 = flat-sequence {
    tunnel: w69 -> [w337]
    tunnel: [w336] -> w68
    tunnel: w67 -> [w335]
    frame #0 {
      n124 = Merge Errors(w335, w337) -> (w336:errorcluster)
      n125 = local write "Stop"(FALSE ("STOP")) -> ()
    }
  }
  n126 = Release Queue(queue=w16, error in (no error)=w15) -> ()  [unwired: 1 in, 3 out]
  n127 = Release Queue(queue=w13, error in (no error)=w12) -> ()  [unwired: 1 in, 3 out]
  n128 = disable-structure shown="Disabled" {
    disable-tunnel: w10 -> [w341 _]
    disable-tunnel: w9 -> [w340 _]
    frame Disabled {
      n129 = local read "Path"() -> (w339:path)
      n130 = String To Path(string="File Name 3") -> (path=w345:path)
      n131 = Build Path(base path=w339, name or relative path=w345) -> (appended path=w342:path)
      n132 = while {
        shift-right: [w361] -> _
        shift-left: _ -> [w362]
        shift-right: [w357] -> _
        shift-left: _ -> [w360]
        shift-right: [w358] -> _
        shift-left: _ -> [w359]
        shift-right: [w355] -> _
        shift-left: enum16{"Initialize", "BuildArray", "Write"}."Initialize" -> [w356]
        tunnel: w342 -> [w354]
        shift-right: [w351] -> _
        shift-left: _ -> [w350]
        shift-right: [w348] -> _
        shift-left: w341 -> [w349]
        shift-right: [w346] -> _
        shift-left: w340 -> [w347]
        stop <- w352 stop-if-true
        n133 = case shown="\"BuildArray\"" w356 {
          tunnel: w362 -> [_ w389 w400]
          tunnel: [dbl[] [] w384 w400] -> w361
          tunnel: w360 -> [_ w388 w399]
          tunnel: w359 -> [_ w387 w398]
          tunnel: [i32[] [] w386 w398] -> w358
          tunnel: [dbl[] [] w385 w399] -> w357
          tunnel: [enum16{"Initialize", "BuildArray", "Write"}."BuildArray" w378 enum16{"Initialize", "BuildArray", "Write"}."Initialize"] -> w355
          tunnel: w354 -> [_ _ w401]
          tunnel: [w365 w377 w396] -> w351
          tunnel: w350 -> [w365 w377 w395]
          tunnel: w349 -> [w364 w375 w394]
          tunnel: [w364 w374 w394] -> w348
          tunnel: w347 -> [w363 w373 w393]
          tunnel: [w363 w371 w393] -> w346
          frame "Initialize", Default {
          }
          frame "BuildArray" {
            n134 = Dequeue Element(queue=w373) -> (queue out=w371:refnum<queue>, element=w372:dbl[])  [unwired: 2 in, 2 out]
            n135 = Dequeue Element(queue=w375) -> (queue out=w374:refnum<queue>, element=w376:dbl[])  [unwired: 2 in, 2 out]
            n136 = local read "sizeNcsDS"() -> (w370:i32)
            n137 = Insert Into Array(array=w389, new element=w376) -> (w384:dbl[])  [unwired: 1 in]
            n138 = Insert Into Array(array=w388, new element=w372) -> (w385:dbl[])  [unwired: 1 in]
            n139 = for {
              N: w370 -> [_]
              shift-right: [w390] -> w386
              shift-left: w387 -> [w391]
              n140 = local read "ECGsample"() -> (w392:i16)
              n141 = Insert Into Array(array=w391, new element=w392) -> (w390:i32[])  [unwired: 1 in]
            }
            n142 = Array Size(array=w384) -> (size(s)=w383:i32)
            "size(s) 4" <- w383
            n143 = Greater?(x=w383, y="maxWrite 2") -> (0:w381:bool)
            n144 = Select(t=enum16{"Initialize", "BuildArray", "Write"}."Write", s=w381, f=enum16{"Initialize", "BuildArray", "Write"}."BuildArray") -> (s? t:f=w378:enum16{"Initialize", "BuildArray", "Write"})
          }
          frame "Write" {
            n145 = Build Array(w400, w399, w398) -> (w397:dbl[][])
            n146 = call "Convert to Dynamic Data2"("2D Array"=w397) -> ("Dynamic Data Type"=w402:dynamicdata)  [unwired: 3 in]
            n147 = call "Data To File"("Signals"=w402, "error in (no error)"=w395, "Filename"=w401) -> ("error out"=w396:errorcluster)  [unwired: 14 in, 2 out]
          }
        }
        n148 = local read "Stop"() -> (w353:bool)
        n149 = Or(x=w351, y=w353) -> (x .or. y?=w352:bool)
      }
    }
    frame Enabled {
    }
  }
  "error IO" <- w68
